vi "3.1 Generate Act Array.vi"() -> (0 "Array":dbl[](array[numeric]))   [LabVIEW 2010]
uses:
  3.0-Global.vi
panel:
  out "Waveform Graph":dbl[](graph)
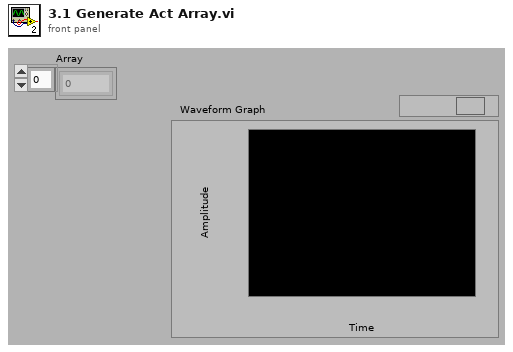
[diagram p1: front panel]
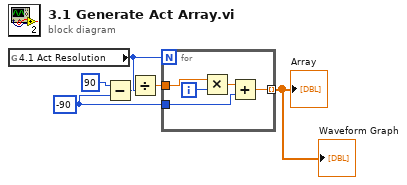
[diagram p0: block diagram]
diagram:
  w5 = -90 ("y")
  n1 = global read "3.0-Global.vi" "4.1 Act Resolution"() -> (w6:u32)
  n2 = Subtract(x=90 ("y"), y=w5) -> (x-y=w3:i32)
  n3 = Divide(x=w3, y=w6) -> (x/y=w4:dbl)
  n4 = for {
    N: w6 -> [_]
    tunnel: w4 -> [w10]
    tunnel: w5 -> [w9]
    tunnel: [w7] -> w1 mode=indexing
    i -> [w8]
    n5 = Multiply(x=w10, y=w8) -> (x*y=w11:dbl)
    n6 = Add(x=w11, y=w9) -> (x+y=w7:dbl)
  }
  "Array" <- w1
  "Waveform Graph" <- w1
